vi "tablica.vi"() -> (3 "array":i32[](array[numeric])=[0, 18, 2, 4, 6, 8, 10, 12, 14, 16, 0, 0, 0, 0, 5, 0, 0, 0, 15, 0, 0, 0, 0, 0, 17, 19, 1, 7, 0, 9, 13, 0, 3, 0, 11])   [LabVIEW 2020]
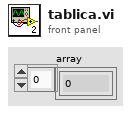
[diagram p1: front panel]
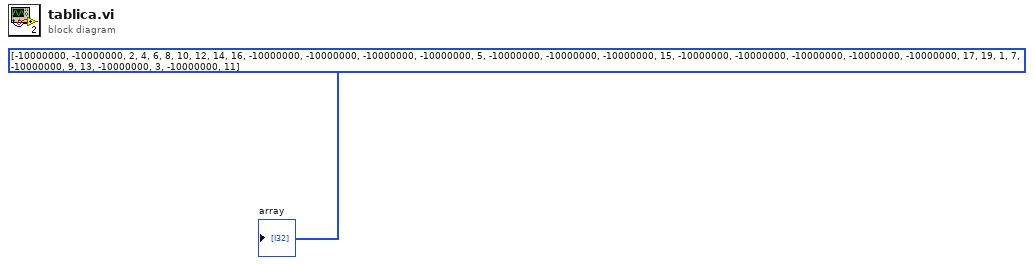
[diagram p0: block diagram]
diagram:
  "array" <- i32[] [-10000000, -10000000, 2, 4, 6, 8, 10, 12, 14, 16, -10000000, -10000000, -10000000, -10000000, 5, -10000000, -10000000, -10000000, 15, -10000000, -10000000, -10000000, -10000000, -10000000, 17, 19, 1, 7, -10000000, 9, 13, -10000000, 3, -10000000, 11] ("array")
